vi "Check Status (No Objects) - Anritsu Power Meter.vi"(8 "error in (no error)":errorcluster, 10 "VISA Resource Name":refnum<visa-resource-name>, 11 "Cluster In":T6={"Averaging"=enum."On", "Units"=enum."Watt", "Measuring rate"=enum."Hold", "Unit Range"=enum."10 mW (+10 dBm)", "Calibration Factor"=-26.67, "Auto Ranging?"=enum."Off"}) -> (0 "error out":errorcluster, 1 "Status":string, 2 "Ready?":bool, 3 "Cluster Out":T6={"Averaging"=enum."On", "Units"=enum."Watt", "Measuring rate"=enum."Hold", "Unit Range"=enum."10 mW (+10 dBm)", "Calibration Factor"=-26.67, "Auto Ranging?"=enum."Off"})   [LabVIEW 2017]
doc: "(Dynamic) Check if the instrument is powered on and update its member fields with the instrument's current status. Optionally return a text status message."
uses:
  Anritsu Power Meter/Public/Averaging control.ctl
  Anritsu Power Meter/Public/Display control.ctl
  Anritsu Power Meter/Public/Measuring rate control.ctl
  Anritsu Power Meter/Public/Range control watts and dBm.ctl
  Anritsu Power Meter/Public/Auto Range control.ctl
  <vilib>/regexp/Match Regular Expression.xnode
  Anritsu Power Meter/Anritsu Power Meter.lvlib
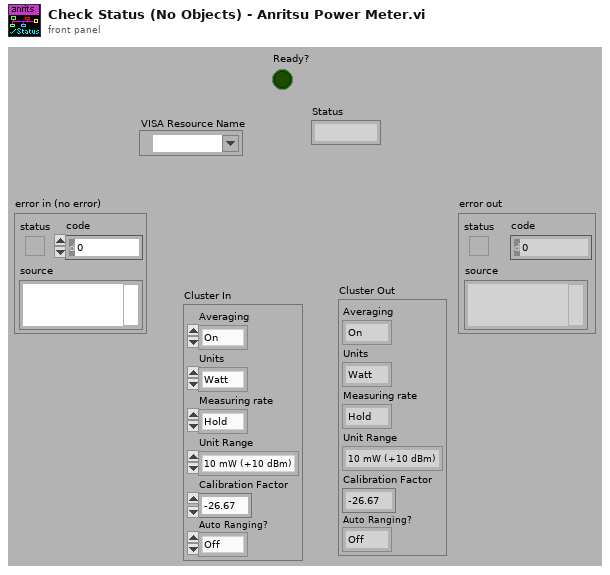
[diagram p1: front panel]
types:
  T1 = typedef "Anritsu Power Meter.lvlib/Averaging control.ctl" = enum16{"On", "Off"}
  T2 = typedef "Anritsu Power Meter.lvlib/Display control.ctl" = enum16{"Watt", "dBm", "dB (REL)"}
  T3 = typedef "Anritsu Power Meter.lvlib/Measuring rate control.ctl" = enum16{"Hold", "Free Run", "Exit Trigger"}
  T4 = typedef "Anritsu Power Meter.lvlib/Range control watts and dBm.ctl" = enum16{"10 mW (+10 dBm)", "1 mW (0 dBm)", "100 uW (-10 dBm)", "10 uW (-20 dBm)", "1 uW (-30 dBm)", "100 nW (-40 dBm)", "10 nW (-50 dBm)", "1 nW (-60 dBm)", "100 pW (-70 dBm)", "10 pW (-80 dBm)"}
  T5 = typedef "Anritsu Power Meter.lvlib/Auto Range control.ctl" = enum16{"Off", "On"}
  T6 = cluster{"Averaging":T1, "Units":T2, "Measuring rate":T3, "Unit Range":T4, "Calibration Factor":dbl, "Auto Ranging?":T5}
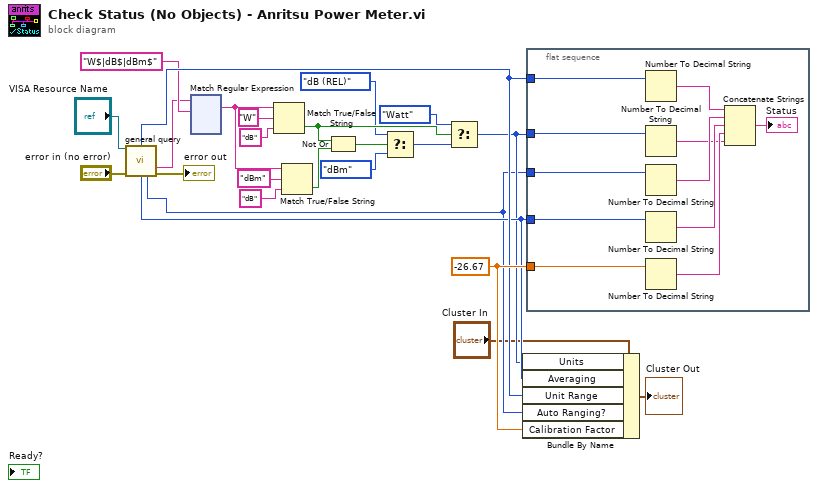
[diagram p0: block diagram]
diagram:
  w24 = -26.67 ("Calibration Factor")
  n1 = call "general query.vi"("VISA resource name"="VISA Resource Name", "error in (no error)"="error in (no error)") -> ("Range W and dBm"=w23:T4, "Units"=w8:string, "Averaging"=w22:T1, "Auto Ranging?"=w6:T5, "error out"=→"error out":errorcluster)  [unwired: 5 in, 4 out]
  n2 = xnode "Match Regular Expression"("input string"=w8, "regular expression"="W$|dB$|dBm$") -> ("whole match"=w18:string)  [unwired: 4 in, 4 out]
  n3 = Match True/False String(2:"dB" ("false string"), 3:"W", 4:w18) -> (0:w14:bool)  [unwired: 1 out]
  n4 = Match True/False String(2:"dB" ("false string"), 3:"dBm" ("true string"), 4:w18) -> (0:w15:bool)  [unwired: 1 out]
  n5 = Not Or(1:w15, 2:w14) -> (0:w12:bool)
  n6 = Select(t=Display_control."dB (REL)" ("Display Units"), s=w12, f=Display_control."dBm" ("Display Units")) -> (s? t:f=w9:T2)
  n7 = Select(t=Display_control."Watt" ("Display Units"), s=w14, f=w9) -> (s? t:f=w7:T2)
  n8 = Bundle By Name(cluster="Cluster In", "Units"=w7, "Averaging"=w22, "Unit Range"=w23, "Auto Ranging?"=w6, "Calibration Factor"=w24) -> (→"Cluster Out":T6)
  n9 = flat-sequence {
    tunnel: w22 -> [w33]
    tunnel: w24 -> [w35]
    tunnel: w7 -> [w32]
    tunnel: w23 -> [w34]
    tunnel: w6 -> [w25]
    frame #0 {
      n10 = Number To Decimal String(number=w34) -> (decimal integer string=w31:string)  [unwired: 1 in]
      n11 = Number To Decimal String(number=w32) -> (decimal integer string=w27:string)  [unwired: 1 in]
      n12 = Number To Decimal String(number=w25) -> (decimal integer string=w30:string)  [unwired: 1 in]
      n13 = Number To Decimal String(number=w33) -> (decimal integer string=w29:string)  [unwired: 1 in]
      n14 = Number To Decimal String(number=w35) -> (decimal integer string=w28:string)  [unwired: 1 in]
      n15 = Concatenate Strings(w31, w30, w29, w28, w27) -> (→"Status":string)
    }
  }
